vi "CONST Default DAQ IO Config.vi"() -> (0 "IO Nodes":T1 {"AO Config"."AO Channels"."Conversion"."ScaleOffset" format="%.3f"; "AO Config"."AO Channels"."Conversion"."MinEngUnit" format="%.3f"; "AO Config"."AO Channels"."Conversion"."MaxEngUnit" format="%.3f"; "AO Config"."AO Channels"."Conversion"."MinSignal" format="%.3f"; "AO Config"."AO Channels"."Conversion"."MaxSignal" format="%.3f"; "AI Config"."AI Tasks"."AI Channels"."Conversion"."ScaleOffset" format="%.3f"; "AI Config"."AI Tasks"."AI Channels"."Conversion"."MinEngUnit" format="%.3f"; "AI Config"."AI Tasks"."AI Channels"."Conversion"."MaxEngUnit" format="%.3f"; "AI Config"."AI Tasks"."AI Channels"."Conversion"."MinSignal" format="%.3f"; "AI Config"."AI Tasks"."AI Channels"."Conversion"."MaxSignal" format="%.3f"; "AI Config"."AI Tasks"."AI Channels"."Terminal Configuration" items=["default"=-1, "RSE"=10083, "NRSE"=10078, "Differential"=10106, "Pseudodifferential"=12529]})   [LabVIEW 2017, in "DAQ.lvclass"]
doc: "Developed by Kevin Thompson\nkevin@thompsonengineering.net\n\nCopyright 2018-2020\nThompson Engineering, LLC"
uses:
  DAQ.lvclass
  DataTypes/TD IO Node Definition--cluster.ctl
  DataTypes/TD DI Config--cluster.ctl
  DataTypes/TD DI Task--cluster.ctl
  DataTypes/TD DI Channel--cluster.ctl
  DataTypes/TD DO Config--cluster.ctl
  DataTypes/TD DO Channel--cluster.ctl
  DataTypes/TD AI Config--cluster.ctl
  DataTypes/TD AI Task--cluster.ctl
  DataTypes/TD AI Channel--cluster.ctl
  DataTypes/TD DataValueConversion--cluster.ctl
  DataTypes/TD AI DAQ Type--enum.ctl
  DataTypes/TD AI Force Bridge--cluster.ctl
  DataTypes/TD AO Config--cluster.ctl
  DataTypes/TD AO Channel--cluster.ctl
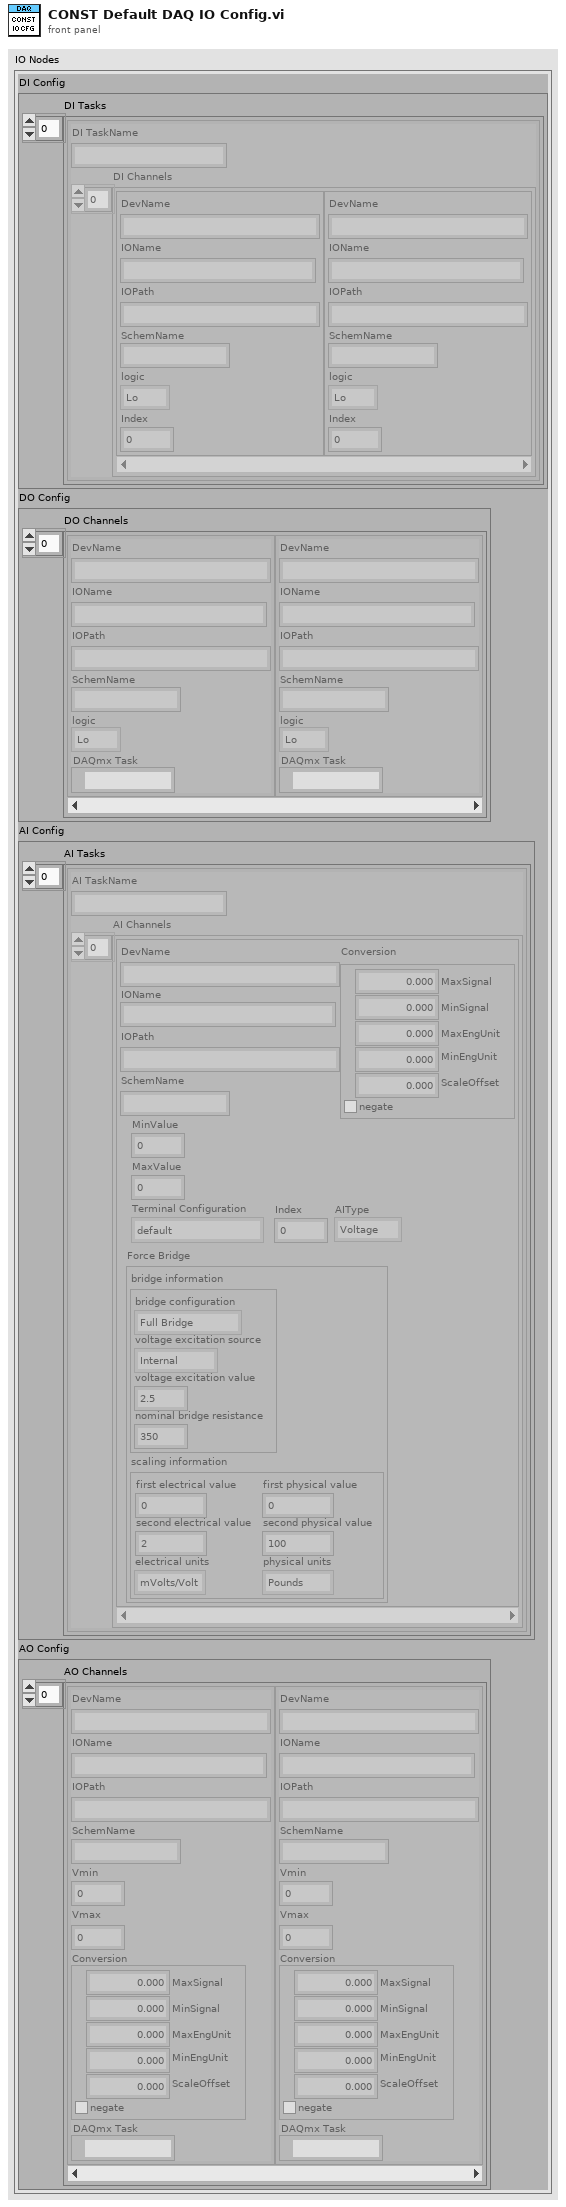
[diagram p1: front panel]
types:
  T1 = typedef "DAQ.lvclass/TD IO Node Definition--cluster.ctl" = cluster{"DI Config":T2, "DO Config":T5, "AI Config":T7, "AO Config":T13}
  T2 = typedef "DAQ.lvclass/TD DI Config--cluster.ctl" = cluster{"DI Tasks":T3[]}
  T3 = typedef "DAQ.lvclass/TD DI Task--cluster.ctl" = cluster{"DI TaskName":string, "DI Channels":T4[]}
  T4 = typedef "DAQ.lvclass/TD DI Channel--cluster.ctl" = cluster{"DevName":string, "IOName":string, "IOPath":string, "SchemName":string, "logic":enum16{"Lo", "Hi"}, "Index":i32}
  T5 = typedef "DAQ.lvclass/TD DO Config--cluster.ctl" = cluster{"DO Channels":T6[]}
  T6 = typedef "DAQ.lvclass/TD DO Channel--cluster.ctl" = cluster{"DevName":string, "IOName":string, "IOPath":string, "SchemName":string, "logic":enum16{"Lo", "Hi"}, "DAQmx Task":refnum<k21>}
  T7 = typedef "DAQ.lvclass/TD AI Config--cluster.ctl" = cluster{"AI Tasks":T8[]}
  T8 = typedef "DAQ.lvclass/TD AI Task--cluster.ctl" = cluster{"AI TaskName":string, "AI Channels":T9[]}
  T9 = typedef "DAQ.lvclass/TD AI Channel--cluster.ctl" = cluster{"DevName":string, "IOName":string, "IOPath":string, "SchemName":string, "MinValue":dbl, "MaxValue":dbl, "Terminal Configuration":i32, "Index":i32, "Conversion":T10, "AIType":T11, "Force Bridge":T12}
  T10 = typedef "DAQ.lvclass/TD DataValueConversion--cluster.ctl" = cluster{"MaxSignal":dbl, "MinSignal":dbl, "MaxEngUnit":dbl, "MinEngUnit":dbl, "ScaleOffset":dbl, "negate":bool}
  T11 = typedef "DAQ.lvclass/TD AI DAQ Type--enum.ctl" = enum16{"Voltage", "Current", "Strain Gage", "Force Bridge"}
  T12 = typedef "DAQ.lvclass/TD AI Force Bridge--cluster.ctl" = cluster{"bridge information":cluster{"bridge configuration":i32, "voltage excitation source":i32, "voltage excitation value":dbl, "nominal bridge resistance":dbl}, "scaling information":cluster{"first electrical value":dbl, "second electrical value":dbl, "electrical units":i32, "first physical value":dbl, "second physical value":dbl, "physical units":i32}}
  T13 = typedef "DAQ.lvclass/TD AO Config--cluster.ctl" = cluster{"AO Channels":T14[]}
  T14 = typedef "DAQ.lvclass/TD AO Channel--cluster.ctl" = cluster{"DevName":string, "IOName":string, "IOPath":string, "SchemName":string, "Vmin":dbl, "Vmax":dbl, "Conversion":T10, "DAQmx Task":refnum<k21>}
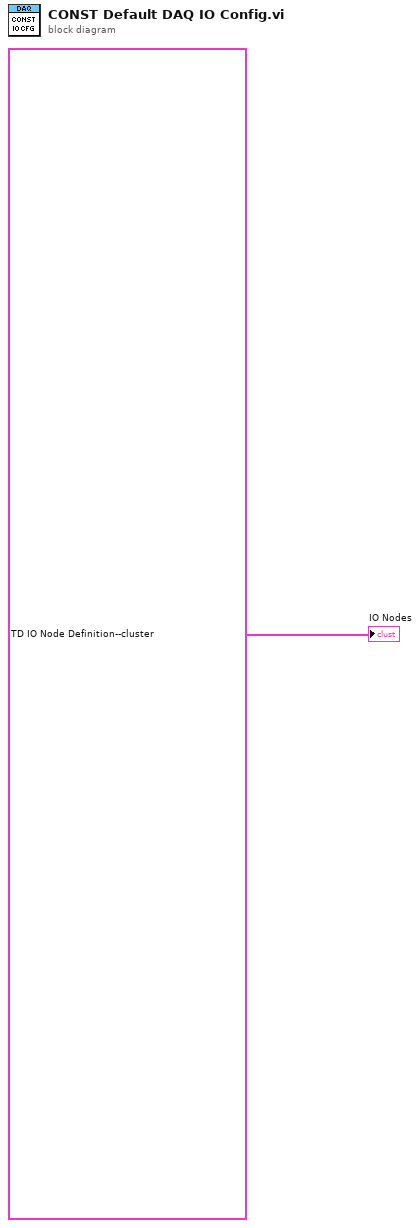
[diagram p0: block diagram]
diagram:
  "IO Nodes" <- T1 {"DI Config"={"DI Tasks"=[{"DI TaskName"="DITask_1", "DI Channels"=[{"DevName"="Mod7-9421", "IOName"="EMO_Signal_DI", "IOPath"="Mod7-9421/port0/Line0", "SchemName"="EMO_Signal", "logic"=enum."Hi", "Index"=0}]}]}, "DO Config"={"DO Channels"=[{"DevName"="Mod4-9482", "IOName"="Relay_0_DO", "IOPath"="Mod4-9482/port0/line0", "SchemName"="CH0", "logic"=enum."Hi", "DAQmx Task"=""}, {"DevName"="Mod4-9482", "IOName"="Relay_1_DO", "IOPath"="Mod4-9482/port0/line1", "SchemName"="CH1", "logic"=enum."Hi", "DAQmx Task"=""}, {"DevName"="Mod4-9482", "IOName"="Relay_2_DO", "IOPath"="Mod4-9482/port0/line2", "SchemName"="CH2", "logic"=enum."Hi", "DAQmx Task"=""}, {"DevName"="", "IOName"="Relay_3_DO", "IOPath"="Mod4-9482/port0/line3", "SchemName"="CH3", "logic"=enum."Hi", "DAQmx Task"=""}]}, "AI Config"={"AI Tasks"=[{"AI TaskName"="AITask_1", "AI Channels"=[{"DevName"="Mod1-9205", "IOName"="DynVoltage_AI", "IOPath"="Mod1-9205/ai0", "SchemName"="DynVoltage", "MinValue"=-10.0, "MaxValue"=10.0, "Terminal Configuration"=10106, "Index"=0, "Conversion"={"MaxSignal"=10.0, "MinSignal"=0.0, "MaxEngUnit"=10.0, "MinEngUnit"=0.0, "ScaleOffset"=0.0, "negate"=FALSE}, "AIType"=enum."Voltage", "Force Bridge"={"bridge information"={"bridge configuration"=0, "voltage excitation source"=0, "voltage excitation value"=0.0, "nominal bridge resistance"=0.0}, "scaling information"={"first electrical value"=0.0, "second electrical value"=0.0, "electrical units"=0, "first physical value"=0.0, "second physical value"=0.0, "physical units"=0}}}, {"DevName"="Mod1-9205", "IOName"="DynCurrent_AI", "IOPath"="Mod1-9205/ai1", "SchemName"="DynCurrent", "MinValue"=-10.0, "MaxValue"=10.0, "Terminal Configuration"=10106, "Index"=0, "Conversion"={"MaxSignal"=10.0, "MinSignal"=0.0, "MaxEngUnit"=10.0, "MinEngUnit"=0.0, "ScaleOffset"=0.0, "negate"=FALSE}, "AIType"=enum."Voltage", "Force Bridge"={"bridge information"={"bridge configuration"=0, "voltage excitation source"=0, "voltage excitation value"=0.0, "nominal bridge resistance"=0.0}, "scaling information"={"first electrical value"=0.0, "second electrical value"=0.0, "electrical units"=0, "first physical value"=0.0, "second physical value"=0.0, "physical units"=0}}}]}]}, "AO Config"={"AO Channels"=[{"DevName"="Mod3-9263", "IOName"="SigOut_1_A0", "IOPath"="Mod3-9263/ao1", "SchemName"="SigOut_1", "Vmin"=-10.0, "Vmax"=10.0, "Conversion"={"MaxSignal"=10.0, "MinSignal"=0.0, "MaxEngUnit"=10.0, "MinEngUnit"=0.0, "ScaleOffset"=0.0, "negate"=FALSE}, "DAQmx Task"=""}, {"DevName"="Mod3-9263", "IOName"="SigOut_2_A0", "IOPath"="Mod3-9263/ao2", "SchemName"="SigOut_2", "Vmin"=-10.0, "Vmax"=10.0, "Conversion"={"MaxSignal"=10.0, "MinSignal"=0.0, "MaxEngUnit"=10.0, "MinEngUnit"=0.0, "ScaleOffset"=0.0, "negate"=FALSE}, "DAQmx Task"=""}, {"DevName"="Mod3-9263", "IOName"="SigOut_3_A0", "IOPath"="Mod3-9263/ao3", "SchemName"="SigOut_3", "Vmin"=-10.0, "Vmax"=10.0, "Conversion"={"MaxSignal"=10.0, "MinSignal"=0.0, "MaxEngUnit"=10.0, "MinEngUnit"=0.0, "ScaleOffset"=0.0, "negate"=FALSE}, "DAQmx Task"=""}]}} ("IO Nodes")
